vi "Create Point Channels.vi"(8 "error in (no error)":errorcluster, 10 "PlayerID":u8, 11 "Parent Ref in":T1 format="%.0x") -> (0 "error out":errorcluster, 3 "Parent Ref out":T1=18446744073709551615 format="%.0x")   [LabVIEW 2023, in "Vires VTD System Explorer.lvlib"]
uses:
  Vires VTD System Explorer.lvlib
  <vilib>/NI VeriStand/Custom Device API/Custom Device Item Ref.ctl
  <vilib>/NI VeriStand/Custom Device API/Custom Device Channel.ctl
  <vilib>/NI VeriStand/Custom Device API/Custom Device Channel Type.ctl
  <vilib>/xnet/xnet.llb/XNET String To IO Name (Frame).vi
  <resource>/objmgr/xnet.rc
  <vilib>/NI VeriStand/Custom Device API/Custom Device API.lvlib
panel:
  out "Name (Short)":string
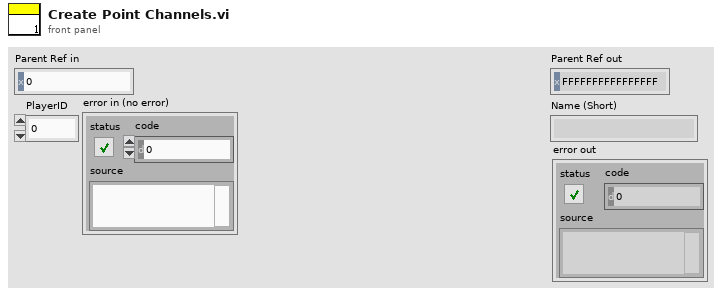
[diagram p1: front panel]
types:
  T1 = typedef "Custom Device API.lvlib/Custom Device Item Ref.ctl" = u64
  T2 = typedef "Custom Device API.lvlib/Custom Device Channel.ctl" = cluster{"Type":T3, "Units":string, "Default Value":dbl, "Faultable":bool, "Scalable":bool}
  T3 = typedef "Custom Device API.lvlib/Custom Device Channel Type.ctl" = enum16{"Input", "Output"}
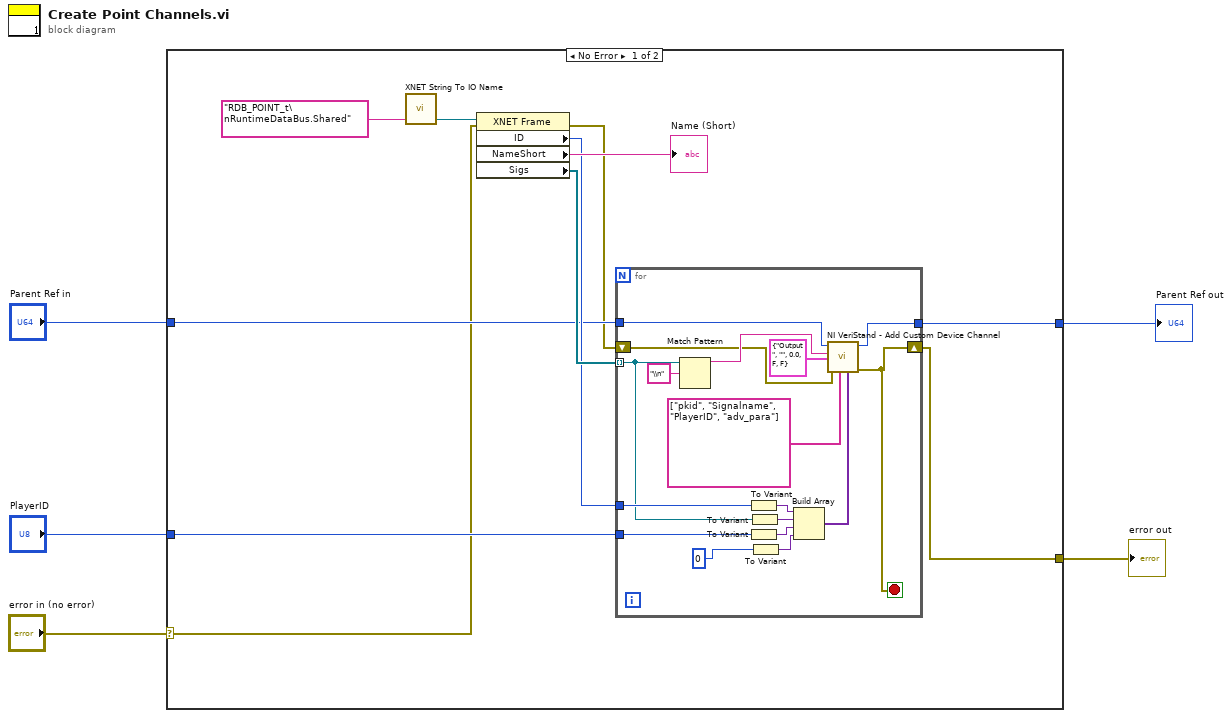
[diagram p0: block diagram]
diagram:
  n1 = case shown="No Error" "error in (no error)" {
    selector: "error in (no error)" -> [w8 w35]
    tunnel: "Parent Ref in" -> [w11 w34]
    tunnel: [w10 w34] -> w4
    tunnel: "PlayerID" -> [w9 _]
    tunnel: [w6 w35] -> w1
    frame No Error {
      n2 = call-poly <vilib>:"XNET String To IO Name.vi"("string"="RDB_POINT_t\nRuntimeDataBus.Shared") -> ("XNET Frame"=w13:refnum<k21>)  [unwired: 4 out]
      n3 = property class="XNET Frame"(reference=w13, error in=w8) -> (error out=w7:errorcluster, "ID"=w12:u32, "NameShort"=→"Name (Short)":string, "Sigs"=w15:refnum<k21>[])  [unwired: 1 out]
      n4 = for {
        tunnel: w15 -> [w24] mode=indexing
        tunnel: w12 -> [w25]
        tunnel: w11 -> [w22]
        tunnel: [w21] -> w10
        tunnel: w9 -> [w20]
        shift-right: [w18] -> w6
        shift-left: w7 -> [w19]
        stop <- w18 stop-if-true
        n5 = Match Pattern(string=w24, regular expression="\\n") -> (before substring=w23:string)  [unwired: 1 in, 3 out]
        n6 = To Variant(anything=w25) -> (Variant=w31:variant)
        n7 = To Variant(anything=w20) -> (Variant=w30:variant)
        n8 = To Variant(anything=w24) -> (Variant=w28:variant)
        n9 = To Variant(anything=0) -> (Variant=w32:variant)
        n10 = Build Array(w31, w28, w30, w32) -> (w29:variant[])
        n11 = call <vilib>:"NI VeriStand - Add Custom Device Channel.vi"("Property Values"=w29, "Property names"=string[] ["pkid", "Signalname", "PlayerID", "adv_para"], "error in (no error)"=w19, "Channel"=T2 {"Type"=enum."Output", "Units"="", "Default Value"=0.0, "Faultable"=FALSE, "Scalable"=FALSE}, "Channel Name"=w23, "Parent Ref in"=w22) -> ("error out"=w18:errorcluster, "Parent Ref out"=w21:T1)  [unwired: 2 in, 2 out]
      }
    }
    frame Error {
    }
  }
  "Parent Ref out" <- w4
  "error out" <- w1
